vi "Blackhawk interfacing.vi"() -> ()   [LabVIEW 2018]
uses:
  <vilib>/Studica/Studica Toolkit/Background/I2C Channel.ctl
  <vilib>/Studica/Studica Blackhawk/Blackhawk.lvlib
panel:
  in  "On/Off":bool
  out "Limit Switch Array":bool[](array[boolean])
  in  "Servo Angle":u8(slide) scale=0.0..180.0
  out "I2C Ref Out":T2
  out "error out":errorcluster
  in  "stop":bool
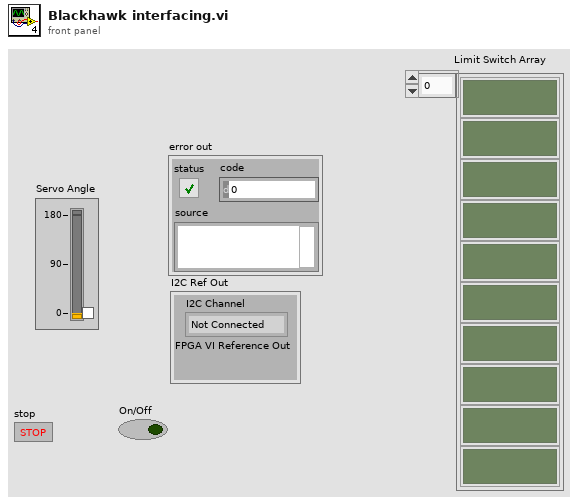
[diagram p1: front panel]
types:
  T1 = typedef "I2C Channel.ctl" = enum16{"Not Connected", "A", "B"}
  T2 = cluster{"I2C Channel":T1, "FPGA VI Reference Out":refnum<k20>}
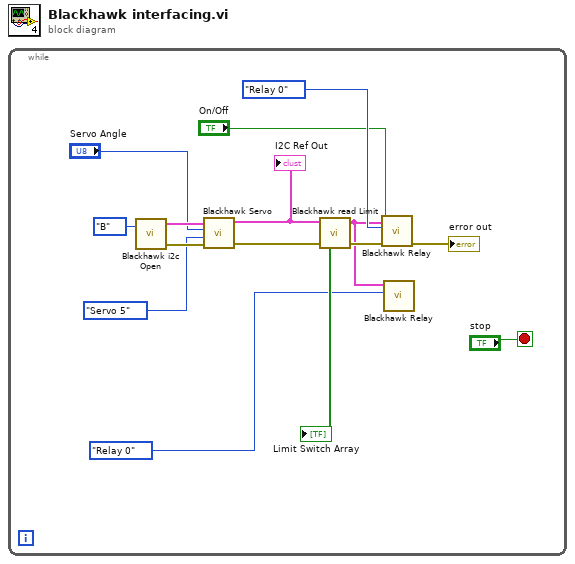
[diagram p0: block diagram]
diagram:
  n1 = while {
    stop <- "stop" stop-if-true
    n2 = call <vilib>:"Blackhawk i2c Open.vi"("I2C Channel"=I2C_Channel."B") -> ("I2C Ref Out"=w13:T2, "error out"=w14:errorcluster)  [unwired: 2 in]
    n3 = call <vilib>:"Blackhawk Servo.vi"("error in (no error)"=w14, "Servo Select"=enum16{"Servo 5", "Servo 6"}."Servo 5", "Servo Angle"="Servo Angle", "I2C Ref In"=w13) -> ("error out"=w6:errorcluster, "I2C Ref Out"=w9:T2)  [unwired: 6 in]
    "I2C Ref Out" <- w9
    n4 = call <vilib>:"Blackhawk read Limit.vi"("error in (no error)"=w6, "I2C Ref In"=w9) -> ("error out"=w7:errorcluster, "Limit Switch Array"=→"Limit Switch Array":bool[], "I2C Ref Out"=w2:T2)  [unwired: 1 in]
    n5 = call <vilib>:"Blackhawk Relay.vi"("error in (no error)"=w7, "On/Off"="On/Off", "Relay"=enum8{"Relay 0", "Relay 1", "Relay 2"}."Relay 0", "I2C Ref In"=w2) -> ("error out"=→"error out":errorcluster)  [unwired: 6 in, 1 out]
    n6 = call <vilib>:"Blackhawk Relay.vi"("Relay"=enum8{"Relay 0", "Relay 1", "Relay 2"}."Relay 0", "I2C Ref In"=w2) -> ()  [unwired: 8 in, 2 out]
  }
